vi "And.vi"() -> ()   [LabVIEW 2019]
panel:
  out "Boolean":bool
  in  "b":bool
  in  "a":bool
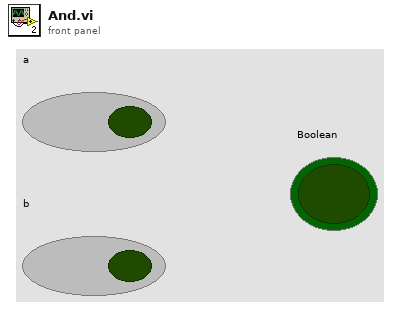
[diagram p1: front panel]
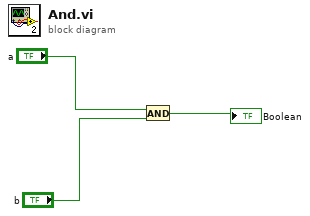
[diagram p0: block diagram]
diagram:
  n1 = And(x="a", y="b") -> (x .and. y?=→"Boolean":bool)
